vi "Transform_Times.vi"(9 "Scalar":dbl, 11 "inTRANSFORM":T1={"TRANSLATION"={"X"=0.0, "Y"=0.0}, "ROTATION"={"VALUE"=0.0, "COS"=1.0, "SIN"=0.0}}) -> (3 "TRANSFORM":T1)   [LabVIEW 2019, in "Trajectory_Library.lvlib"]
doc: "Scales the transform by the scalar.\n\nParameters:\n - IN TRANSFORM - This TRANSFORM data structure\n - SCALAR - The scalar value to multiply the transform by\n\nResults:\n - OUT TRANSFORM - The multiplied transform data structure"
uses:
  Trajectory_Library.lvlib
  TRANSFORM2D.ctl
  TRANSLATION2D.ctl
  ROTATION2D.ctl
  Rotation_CreateAngle.vi
  Translation_Create.vi
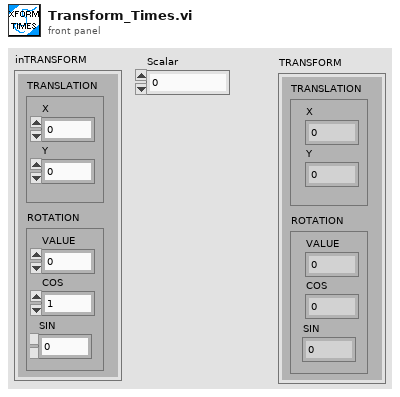
[diagram p1: front panel]
types:
  T1 = typedef "Trajectory_Library.lvlib/TRANSFORM2D.ctl" = cluster{"TRANSLATION":T2, "ROTATION":T3}
  T2 = typedef "Trajectory_Library.lvlib/TRANSLATION2D.ctl" = cluster{"X":dbl, "Y":dbl}
  T3 = typedef "Trajectory_Library.lvlib/ROTATION2D.ctl" = cluster{"VALUE":dbl, "COS":dbl, "SIN":dbl}
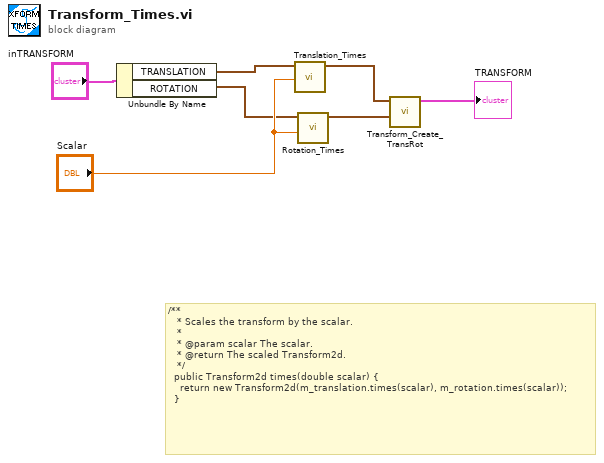
[diagram p0: block diagram]
diagram:
  # "/**\n   * Scales the transform by the scalar.\n   *\n   * @param scalar The scalar.\n   * @return The scaled Transform2d.\n   */\n  public Transform2d times(double scalar) {\n    return new Transform2d(m_translation.times(scalar), m_rotation.times(scalar));\n  }"
  n1 = Unbundle By Name("inTRANSFORM") -> ("TRANSLATION"=w5:T2, "ROTATION"=w2:T3)
  n2 = call "Translation_Times.vi"("Scalar"="Scalar", "In Translation"=w5) -> ("Out Translation"=w4:T2)  [unwired: 9 in]
  n3 = call "Rotation_Times.vi"("Scalar"="Scalar", "in ROTATION"=w2) -> ("out ROTATION"=w1:T3)  [unwired: 9 in]
  n4 = call "Transform_Create_TransRot.vi"("ROTATION"=w1, "TRANSLATION"=w4) -> ("TRANSFORM"=→"TRANSFORM":T1)  [unwired: 9 in]
